vi "Offset_decoder_CH1_no_sign.vi"(11 "Array In1":i8[](array[numeric])) -> (3 "CH1":dbl)   [LabVIEW 2012]
panel:
  out "CH1 3":u8 format="%x"
  out "CH1 2":u8 format="%x"
  out "CH1 1":u8 format="%x"
  out "CH1 0":u8 format="%x"
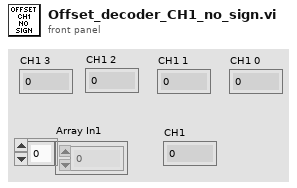
[diagram p1: front panel]
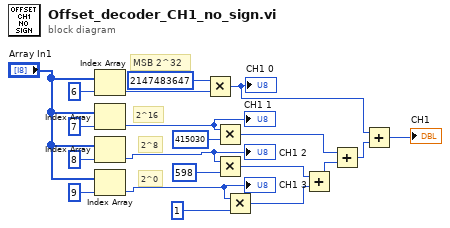
[diagram p0: block diagram]
diagram:
  # "2^0"
  # "2^8"
  # "2^16"
  # "MSB 2^32"
  n1 = Index Array(array="Array In1", index=6) -> (element=w2:i8)
  n2 = Index Array(array="Array In1", index=7) -> (element=w8:i8)
  "CH1 1" <- w8
  n3 = Index Array(array="Array In1", index=8) -> (element=w6:i8)
  "CH1 2" <- w6
  n4 = Index Array(array="Array In1", index=9) -> (element=w7:i8)
  "CH1 3" <- w7
  n5 = Multiply(x=2147483647, y=w2) -> (x*y=w3:i32)
  "CH1 0" <- w3
  n6 = Multiply(x=w8, y=415030) -> (x*y=w10:i32)
  n7 = Multiply(x=w6, y=598) -> (x*y=w13:i32)
  n8 = Multiply(x=w7, y=1) -> (x*y=w12:i32)
  n9 = Add(x=w13, y=w12) -> (x+y=w11:i32)
  n10 = Add(x=w10, y=w11) -> (x+y=w9:i32)
  n11 = Add(x=w3, y=w9) -> (x+y=→"CH1":i32)
